vi "Torros_Slnd.vi"(11 "Toggle?":bool) -> (0 "CurrState":bool)   [LabVIEW 2018]
uses:
  <vilib>/Rock Robotics/WPI/Solenoid/Deprecated/WPI_SolenoidSetBool.vi
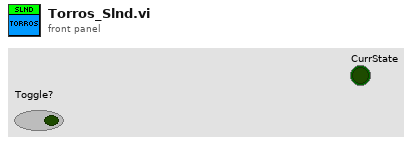
[diagram p1: front panel]
types:
  T1 = typedef "WPI_SolenoidDevRef.ctl" = cluster{"DevStatus":errorcluster, "Pneumatics Control Module":u8, "Forward Solenoid Channel":T2, "Reverse Solenoid Channel":T2}
  T2 = typedef "WPI_SolenoidChannel.ctl" = enum8{"Solenoid 0", "Solenoid 1", "Solenoid 2", "Solenoid 3", "Solenoid 4", "Solenoid 5", "Solenoid 6", "Solenoid 7", "Invalid"}
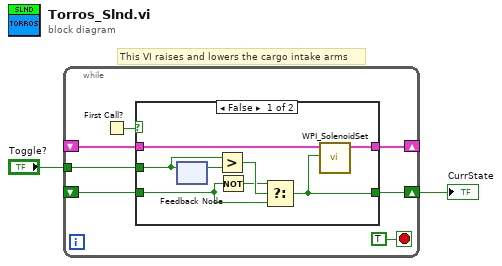
[diagram p0: block diagram]
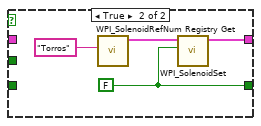
[diagram p2: hidden frame]
diagram:
  # "This VI raises and lowers the cargo intake arms"
  n1 = while {
    shift-right: [w9] -> _
    shift-left: _ -> [w7]
    tunnel: "Toggle?" -> [w8]
    shift-right: [w6] -> w1
    shift-left: _ -> [w5]
    stop <- TRUE stop-if-true
    n2 = First Call?() -> (First Call?: T/F=w3:bool)
    n3 = case shown="False" w3 {
      tunnel: [w17 w19] -> w9
      tunnel: w8 -> [w15 _]
      tunnel: w7 -> [w14 _]
      tunnel: [w13 w18] -> w6
      tunnel: w5 -> [w10 _]
      frame False {
        n4 = feedback #1() -> (w16:bool)  [unwired: 1 in]
        n5 = feedback-in #1(w15) -> ()
        n6 = Greater?(x=w15, y=w16) -> (0:w12:bool)
        n7 = Not(x=w10) -> (.not. x?=w11:bool)
        n8 = Select(t=w11, s=w12, f=w10) -> (s? t:f=w13:bool)
        n9 = call-poly <vilib>:"WPI_SolenoidSet.vi"("Value"=w13, "SolenoidDevRef"=w14) -> ("SolenoidDevRef"=w17:T1)  [unwired: 8 in, 1 out]
      }
      frame True {
        w18 = FALSE
        n10 = call <vilib>:"WPI_SolenoidRefNum Registry Get.vi"("refnum name"="Torros") -> ("SolenoidDevRef"=w20:T1)  [unwired: 9 in, 1 out]
        n11 = call-poly <vilib>:"WPI_SolenoidSet.vi"("Value"=w18, "SolenoidDevRef"=w20) -> ("SolenoidDevRef"=w19:T1)  [unwired: 8 in, 1 out]
      }
    }
  }
  "CurrState" <- w1
